vi "Initialize Interpreter.vi"(8 "error in (no error)":errorcluster) -> (0 "error out":errorcluster, 3 "Already Initialized":bool)   [LabVIEW 2020, in "G-Embedded-Python-Interpreter-Toolkit.lvlib"]
uses:
  G-Embedded-Python-Interpreter-Toolkit.lvlib
  bin/gepit.cp310.32.dll
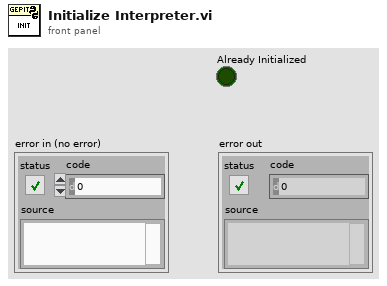
[diagram p1: front panel]
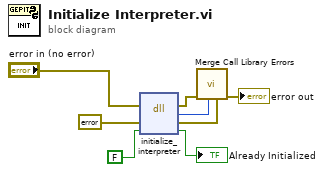
[diagram p0: block diagram]
diagram:
  n1 = dll-call lib="C:/serenial/libraries/g-embedded-python-interpreter-toolkit/LabVIEW/bin/gepit.cp310.32.dll" fn="initialize_interpreter"(error in="error in (no error)", "Error"=errorcluster {"status"=FALSE, "code"=0, "source"=""} ("error constant"), "Already Initialized"=FALSE) -> (error out=w3:errorcluster, "return type"=w2:i32, "Error"=w1:errorcluster, "Already Initialized"=→"Already Initialized":bool)  [unwired: 2 in, 1 out]
  n2 = call "Merge Call Library Errors.vi"("Call Library Error"=w1, "Return Value"=w2, "error in"=w3) -> ("error out"=→"error out":errorcluster)  [unwired: 8 in]
